vi "OnClick.vi"(0 "reference in":refnum<class "Button.lvclass">, 11 "Error In":errorcluster) -> (4 "reference out":refnum<class "Button.lvclass">, 15 "Error Out":errorcluster)   [LabVIEW 2024, in "Button.lvclass"]
uses:
  Button.lvclass
  Button.lvclass/Button.ctl
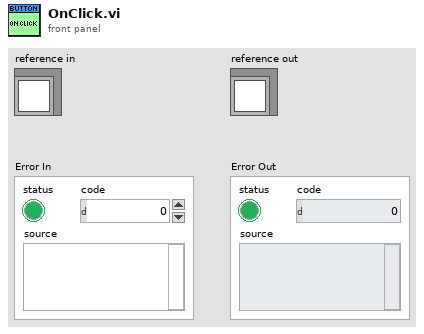
[diagram p1: front panel]
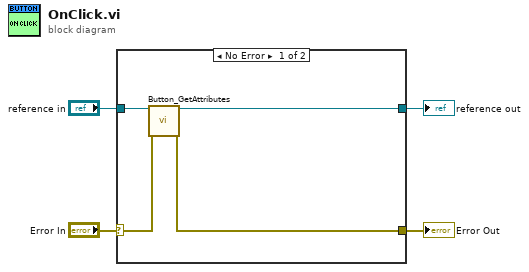
[diagram p0: block diagram]
diagram:
  n1 = case shown="No Error" "Error In" {
    selector: "Error In" -> [w8 w10]
    tunnel: [w7 w10] -> w3
    tunnel: [w5 w9] -> w1
    tunnel: "reference in" -> [w6 w9]
    frame No Error {
      n2 = call "Button_GetAttributes.vi"("reference in"=w6, "Error In"=w8) -> ("reference out"=w5:refnum<class "Button.lvclass">, "Error Out"=w7:errorcluster)  [unwired: 10 in, 2 out]
    }
    frame Error {
    }
  }
  "Error Out" <- w3
  "reference out" <- w1
